vi "mlink_ai_scan_stop (to change).vi"(8 "error in (no error)":errorcluster, 11 "connection ID":i32=-1) -> (0 "error out":errorcluster, 3 "connection ID out":i32)   [LabVIEW 2009, in "MicroDAQ.lvlib" / "mlink.lvlib"]
doc: "This function stops analog input acquisition. Function can be used to interrupt acquisition when scanning session initialized with duration > 0, or to stop continuous acquisition when scanning session initialized with duration = -1 . After calling mlink_ai_scan_stop() function scanning session has to be re-initialized."
uses:
  <instrlib>/MicroDAQ/Mlink library wraper/mlink.lvlib
  <instrlib>/MicroDAQ/MLink32.dll
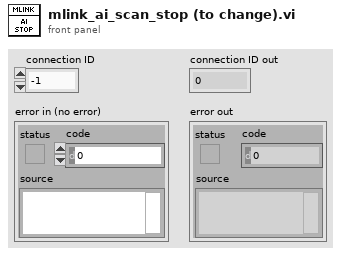
[diagram p1: front panel]
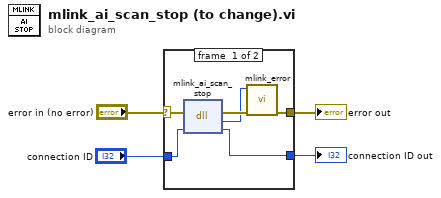
[diagram p0: block diagram]
diagram:
  n1 = case shown="No Error" "error in (no error)" {
    selector: "error in (no error)" -> [w10 w12]
    tunnel: [w8 w12] -> w3
    tunnel: "connection ID" -> [w6 w11]
    tunnel: [w5 w11] -> w1
    frame #0 {
      n2 = dll-call lib="C:/Program Files (x86)/National Instruments/LabVIEW 2009/instr.lib/MicroDAQ/MLink32.dll" fn="mlink_ai_scan_stop"(error in=w10, "link_fd"=w6) -> (error out=w9:errorcluster, "return type"=w7:i32, "link_fd"=w5:i32)  [unwired: 2 in, 1 out]
      n3 = call <instrlib>:"mlink_error.vi"("error in (no error)"=w9, "error code"=w7) -> ("error out"=w8:errorcluster)  [unwired: 9 in]
    }
    frame #1 {
    }
  }
  "error out" <- w3
  "connection ID out" <- w1
